vi "bit-array-to-payload.vi"(4 "Array":bool[](array[boolean])) -> (1 "payload":u8[](array[numeric]) format="%02x")   [LabVIEW 2015]
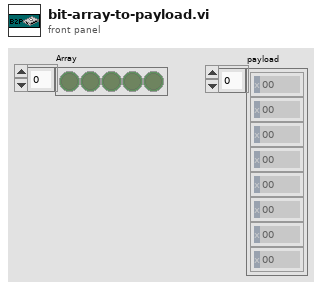
[diagram p1: front panel]
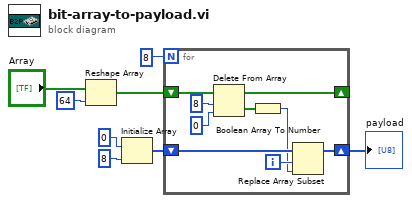
[diagram p0: block diagram]
diagram:
  n1 = Reshape Array("Array", 64 ("dimension size")) -> (w5:bool[])
  n2 = Initialize Array(u8 0, 8 ("dimension size")) -> (w3:u8[])
  n3 = for {
    N: 8 -> [_]
    shift-right: [w15] -> _
    shift-left: w5 -> [w17]
    shift-right: [w12] -> w4
    shift-left: w3 -> [w13]
    i -> [w11]
    n4 = Delete From Array(array=w17, length=8, index=0) -> (deleted portion=w14:bool[], array with subset deleted=w15:bool[])
    n5 = Boolean Array To Number(Boolean array=w14) -> (number=w10:u32)
    n6 = Replace Array Subset(array=w13, new element=w10, index=w11) -> (w12:u8[])
  }
  "payload" <- w4
